vi "Get User Input.vi"(0 "Window Title":string, 7 "Dialog Message":string, 11 "Error In":errorcluster) -> (4 "User Input":string, 8 "Canceled?":bool, 15 "Error Out":errorcluster)   [LabVIEW 2020]
uses:
  <vilib>/Utility/miscctls.llb/LVPointTypeDef.ctl
  <vilib>/Utility/error.llb/whitespace.ctl
panel:
  in  "Get User Input":string caption="Yap Yap"
  in  "Cancel":bool
  in  "Done":bool
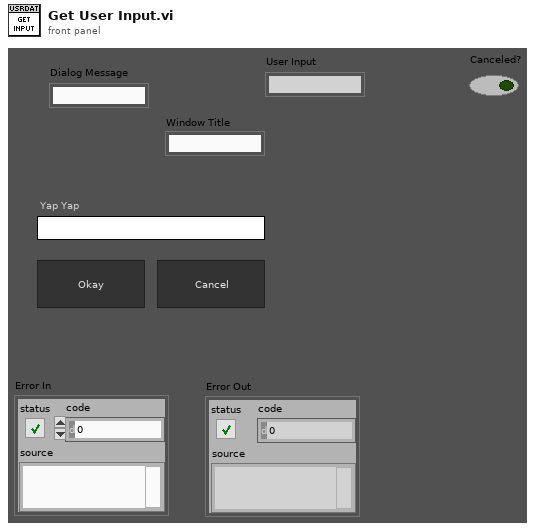
[diagram p1: front panel]
types:
  T1 = enum16{"Always On", "Always Off", "Off While Running"}
  T2 = typedef "LVPointTypeDef.ctl" = cluster{"Horizontal":i16, "Vertical":i16}
  T3 = typedef "LVRectTypeDef.ctl" = cluster{"Left":i16, "Top":i16, "Right":i16, "Bottom":i16}
  T4 = typedef "LVBoundsTypeDef.ctl" = cluster{"Width":u32, "Height":u32}
  T5 = typedef "whitespace.ctl" = u16
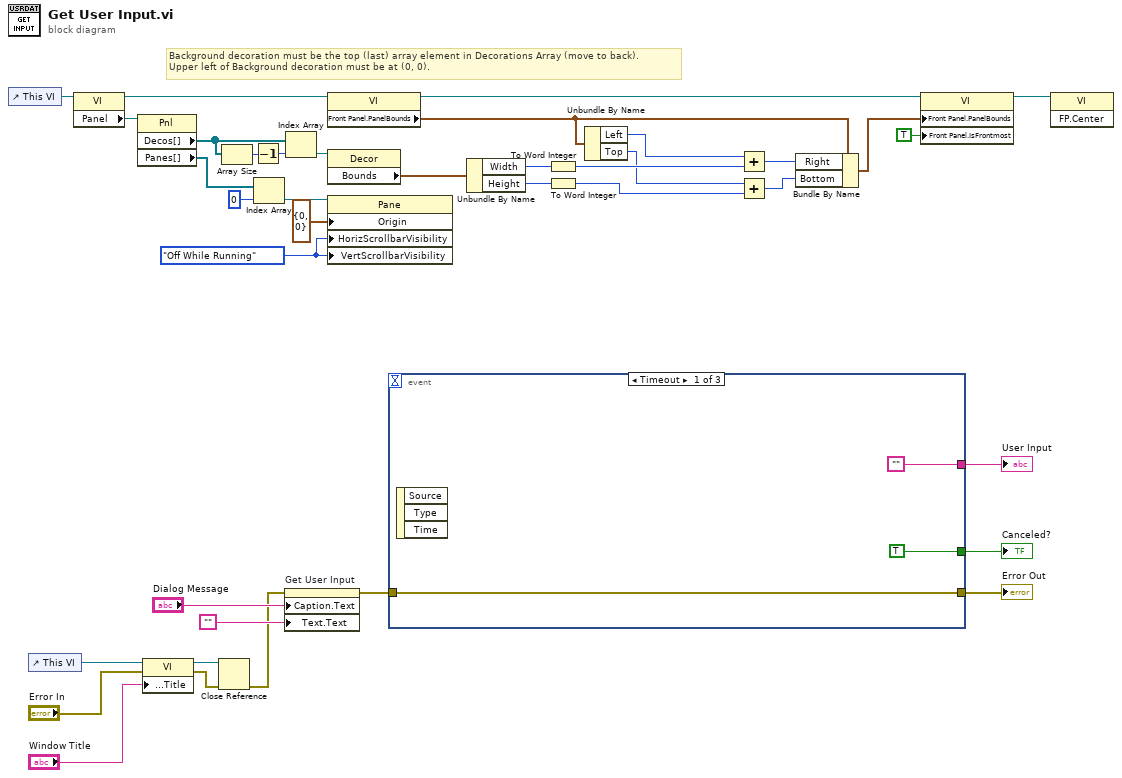
[diagram p0: block diagram]
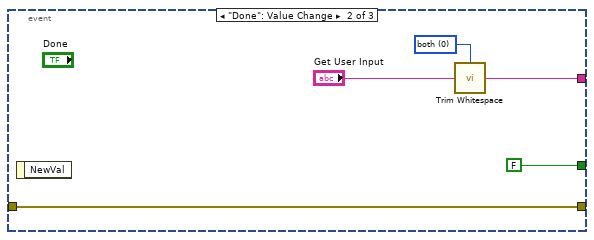
[diagram p2: hidden frame]
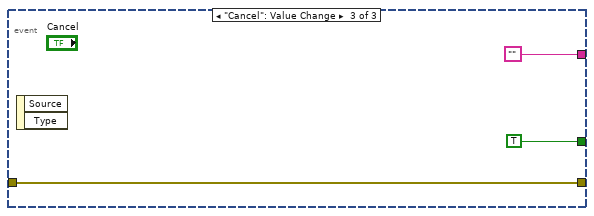
[diagram p3: hidden frame]
diagram:
  w28 = T1."Off While Running" ("Vertical Scrollbar Visibility")
  # "Background decoration must be the top (last) array element in Decorations Array (move to back).\nUpper left of Background decoration must be at (0, 0)."
  n1 = control-ref of="This VI"() -> (w21:refnum<vi>)
  n2 = control-ref of="This VI"() -> (w11:refnum<vi>)
  n3 = property class="VI"(reference=w21) -> (reference out=w29:refnum<vi>, "Panel"=w22:refnum<vi>)  [unwired: 1 in, 1 out]
  n4 = property class="Pnl"(reference=w22) -> ("Decos[]"=w20:refnum<vi>[], "Panes[]"=w25:refnum<vi>[])  [unwired: 1 in, 2 out]
  n5 = property class="VI"(reference=w11, error in="Error In", "Front Panel.Title"="Window Title") -> (reference out=w8:refnum<vi>, error out=w7:errorcluster)
  n6 = Close Reference(reference=w8, error in (no error)=w7) -> (error out=w6:errorcluster)
  n7 = Array Size(array=w20) -> (size(s)=w18:i32)
  n8 = Decrement(x=w18) -> (x-1=w19:i32)
  n9 = Index Array(array=w25, index=0) -> (element=w24:refnum<vi>)
  n10 = property on="Get User Input" class="Str"(error in=w6, "Caption.Text"="Dialog Message", "Text.Text"="") -> (error out=w2:errorcluster)  [unwired: 1 in, 1 out]
  n11 = Index Array(array=w20, index=w19) -> (element=w27:refnum<vi>)
  n12 = property class="VI"(reference=w29) -> (reference out=w31:refnum<vi>, "Front Panel.PanelBounds"=w32:T3)  [unwired: 1 in, 1 out]
  n13 = property class="Decor"(reference=w27) -> ("Bounds"=w30:T4)  [unwired: 1 in, 2 out]
  n14 = property class="Pane"(reference=w24, "Origin"=T2 {"Horizontal"=0, "Vertical"=0}, "HorizScrollbarVisibility"=w28, "VertScrollbarVisibility"=w28) -> ()  [unwired: 1 in, 2 out]
  n15 = event shown="[0] Timeout" {
    selector: _ -> [_ _ _]
    dyn-events: _ -> [_ _ _]
    timeout: _ -> [_ _ _]
    tunnel: ["" w44 ""] -> w14
    tunnel: [TRUE FALSE TRUE] -> w13
    tunnel: w2 -> [w39 w42 w47]
    tunnel: [w39 w42 w47] -> w1
    event Timeout {
      n16 = event-data() -> ()  [unwired: 1 in, 3 out]
    }
    event "Done": Value Change {
      w43 = T5 0 items=["both", "start of string", "end of string"] ("location (both)")
      n17 = event-data() -> ()  [unwired: 1 in, 1 out]
      n18 = call <vilib>:"Trim Whitespace.vi"("string"="Get User Input", "location (both)"=w43) -> ("trimmed string"=w44:string)
    }
    event "Cancel": Value Change {
      n19 = event-data() -> ()  [unwired: 1 in, 2 out]
    }
  }
  "Canceled?" <- w13
  "User Input" <- w14
  "Error Out" <- w1
  n20 = Unbundle By Name(w30) -> ("Width"=w35:u32, "Height"=w38:u32)
  n21 = To Word Integer(number=w35) -> (16bit integer=w37:i16)
  n22 = To Word Integer(number=w38) -> (16bit integer=w3:i16)
  n23 = Unbundle By Name(w32) -> ("Left"=w34:i16, "Top"=w5:i16)
  n24 = Add(x=w34, y=w37) -> (x+y=w36:i16)
  n25 = Add(x=w5, y=w3) -> (x+y=w4:i16)
  n26 = Bundle By Name(cluster=w32, "Right"=w36, "Bottom"=w4) -> (w33:T3)
  n27 = property class="VI"(reference=w31, "Front Panel.PanelBounds"=w33, "Front Panel.IsFrontmost"=TRUE ("Front Panel Window:Is Frontmost")) -> (reference out=w16:refnum<vi>)  [unwired: 1 in, 1 out]
  n28 = invoke class="VI" method="FP.Center"(reference=w16) -> ()  [unwired: 2 in, 3 out]
